vi "Check and Move Files.vi"(8 "error in":errorcluster) -> (0 "error out":errorcluster)   [LabVIEW 2026, in "WebPage Addon Engine.lvlib"]
uses:
  WebPage Addon Engine.lvlib
panel:
  out "file or folder exists?":bool
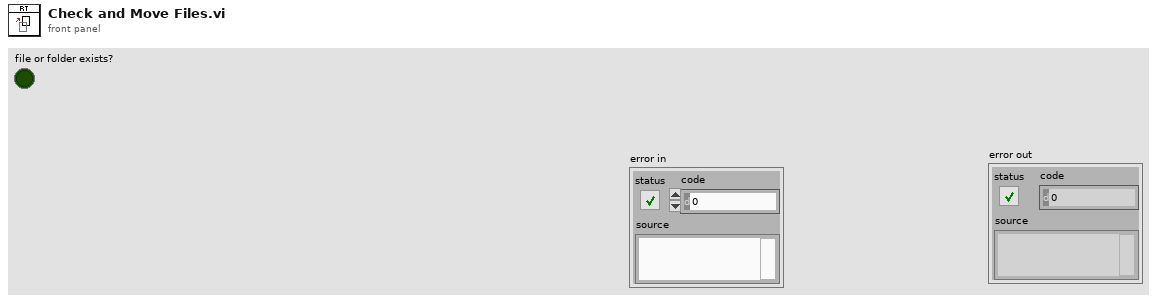
[diagram p1: front panel]
types:
  T1 = cluster{"Source Folder":path, "Target Folder":path, "File":string}[]
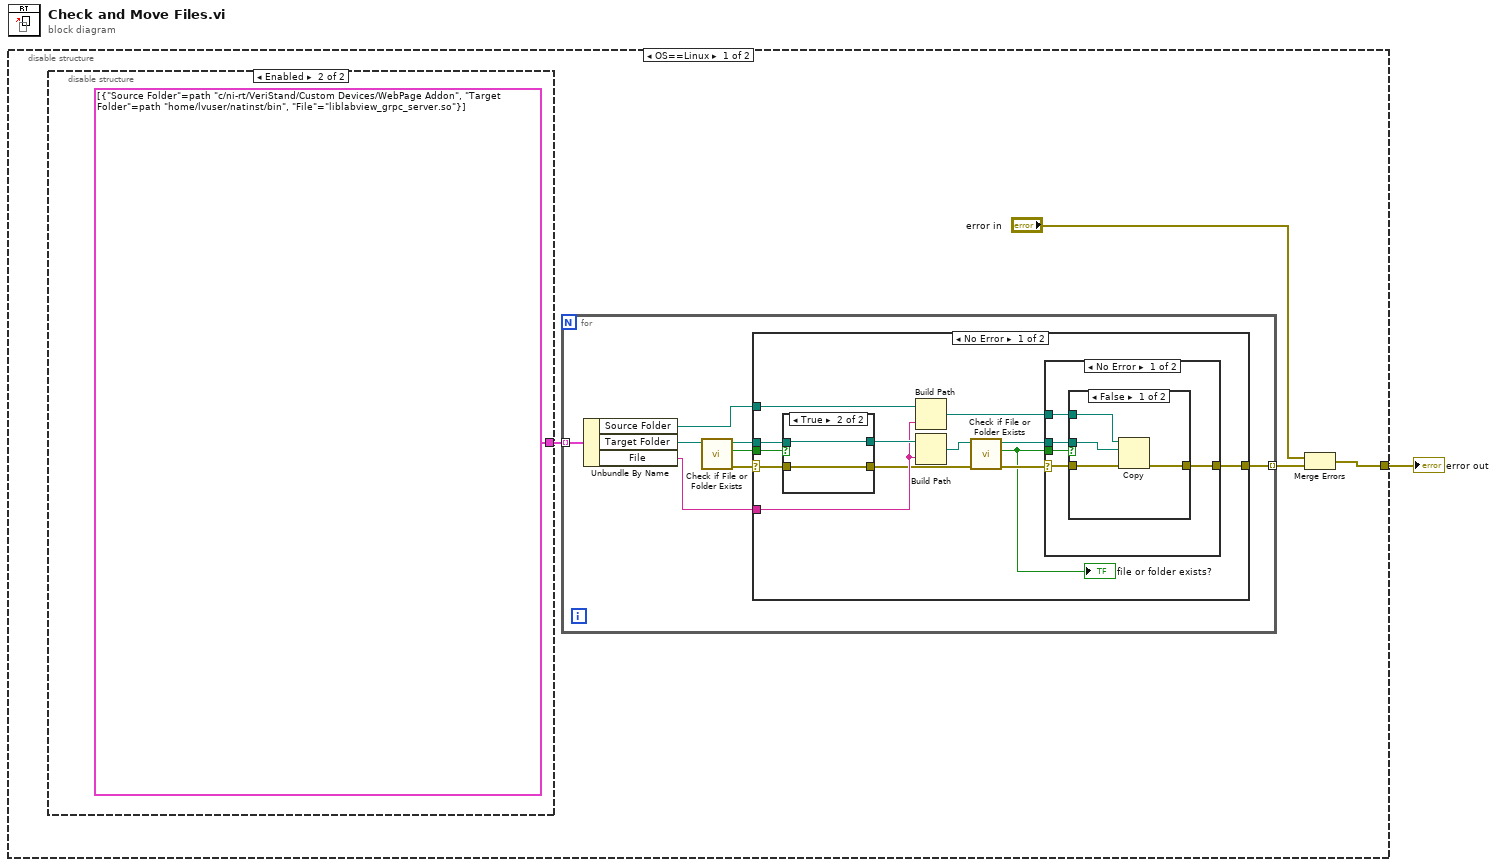
[diagram p0: block diagram]
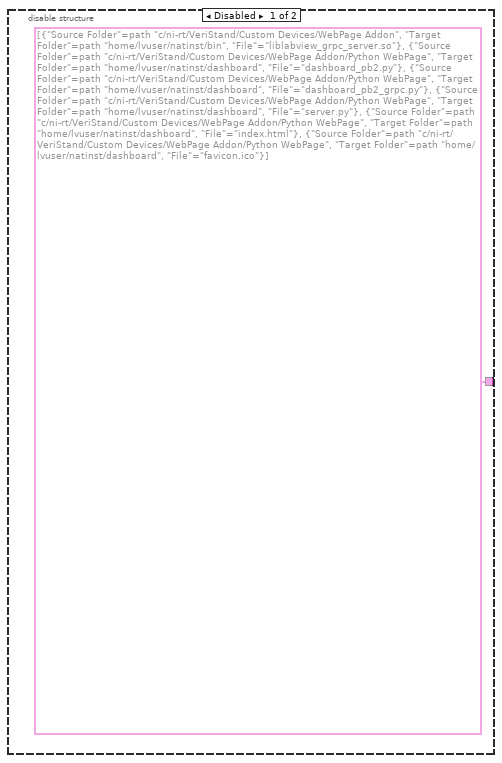
[diagram p2: hidden frame]
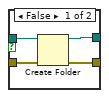
[diagram p3: hidden frame]
diagram:
  n1 = disable-structure shown="OS==Linux" {
    disable-tunnel: [w3 _] -> w1
    frame condition #0 (active) {
      n2 = disable-structure shown="Enabled" {
        disable-tunnel: [T1 [{"Source Folder"=path "c:/ni-rt/VeriStand/Custom Devices/WebPage Addon", "Target Folder"=path "/home/lvuser/natinst/bin", "File"="liblabview_grpc_server.so"}, {"Source Folder"=path "c:/ni-rt/VeriStand/Custom Devices/WebPage Addon/Python WebPage", "Target Folder"=path "/home/lvuser/natinst/dashboard", "File"="dashboard_pb2.py"}, {"Source Folder"=path "c:/ni-rt/VeriStand/Custom Devices/WebPage Addon/Python WebPage", "Target Folder"=path "/home/lvuser/natinst/dashboard", "File"="dashboard_pb2_grpc.py"}, {"Source Folder"=path "c:/ni-rt/VeriStand/Custom Devices/WebPage Addon/Python WebPage", "Target Folder"=path "/home/lvuser/natinst/dashboard", "File"="server.py"}, {"Source Folder"=path "c:/ni-rt/VeriStand/Custom Devices/WebPage Addon/Python WebPage", "Target Folder"=path "/home/lvuser/natinst/dashboard", "File"="index.html"}, {"Source Folder"=path "c:/ni-rt/VeriStand/Custom Devices/WebPage Addon/Python WebPage", "Target Folder"=path "/home/lvuser/natinst/dashboard", "File"="favicon.ico"}] T1 [{"Source Folder"=path "c:/ni-rt/VeriStand/Custom Devices/WebPage Addon", "Target Folder"=path "/home/lvuser/natinst/bin", "File"="liblabview_grpc_server.so"}]] -> w4
        frame Disabled {
        }
        frame Enabled {
        }
      }
      n3 = for {
        tunnel: [w15] -> w5 mode=indexing
        tunnel: w4 -> [w14] mode=indexing
        n4 = Unbundle By Name(w14) -> ("Source Folder"=w8:path, "Target Folder"=w13:path, "File"=w9:string)
        n5 = call <vilib>:"Check if File or Folder Exists.vi"("path"=w13) -> ("error out"=w10:errorcluster, "file or folder exists?"=w12:bool, "dup path"=w11:path)  [unwired: 8 in]
        n6 = case shown="No Error" w10 {
          selector: w10 -> [w20 w46]
          tunnel: [w23 w46] -> w15
          tunnel: w12 -> [w22 _]
          tunnel: w11 -> [w21 _]
          tunnel: w9 -> [w18 _]
          tunnel: w8 -> [w17 _]
          frame No Error {
            n7 = case shown="True" w22 {
              tunnel: w20 -> [w31 w34]
              tunnel: w21 -> [w32 w33]
              tunnel: [w30 w34] -> w16
              tunnel: [w29 w33] -> w19
              frame False {
                n8 = Create Folder(path (use dialog)=w32, error in=w31) -> (created path=w29:path, error out=w30:errorcluster)  [unwired: 1 in, 1 out]
              }
              frame True {
              }
            }
            n9 = Build Path(base path=w17, name or relative path=w18) -> (appended path=w24:path)
            n10 = Build Path(base path=w19, name or relative path=w18) -> (appended path=w28:path)
            n11 = call <vilib>:"Check if File or Folder Exists.vi"("error in (no error)"=w16, "path"=w28) -> ("error out"=w27:errorcluster, "file or folder exists?"=w26:bool, "dup path"=w25:path)  [unwired: 7 in]
            "file or folder exists?" <- w26
            n12 = case shown="No Error" w27 {
              selector: w27 -> [w38 w45]
              tunnel: w26 -> [w39 _]
              tunnel: w25 -> [w37 _]
              tunnel: w24 -> [w36 _]
              tunnel: [w35 w45] -> w23
              frame No Error {
                n13 = case shown="False" w39 {
                  tunnel: w38 -> [w43 w44]
                  tunnel: w37 -> [w42 _]
                  tunnel: w36 -> [w41 _]
                  tunnel: [w40 w44] -> w35
                  frame False {
                    n14 = Copy(8:w43, 10:w42, 11:w41) -> (0:w40:errorcluster)  [unwired: 2 in, 2 out]
                  }
                  frame True {
                  }
                }
              }
              frame Error {
              }
            }
          }
          frame Error {
          }
        }
      }
      n15 = Merge Errors("error in", w5) -> (w3:errorcluster)
    }
    frame condition #1 {
    }
  }
  "error out" <- w1
